vi "Get Target Temperature.vi"   [LabVIEW 2013, in "LMH-Nest.lvlib"]
doc: "Get the target temperature of the specified Nest device."
uses:
  LMH-Nest.lvlib
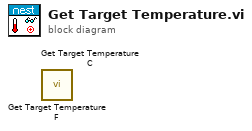
[diagram p0: block diagram]
diagram:
  n1 = call "Get Target Temperature F.vi"() -> ()  [unwired: 7 in, 5 out]
  n2 = call "Get Target Temperature C.vi"() -> ()  [unwired: 7 in, 5 out]
